vi "Parse EST Clusters into EST IP - Multi FPGA.vi"(8 "error in (no error)":errorcluster, 9 "RIO device address":string, 10 "EST version enum":T2, 11 "EPS IP LUT":variant) -> (0 "error out":errorcluster, 2 "Properties":T1[](array[typedef]), 3 "APUs":string[](array[string]))   [LabVIEW 2015, in "Engine Simulation Toolkit System Explorer.lvlib"]
uses:
  Engine Simulation Toolkit System Explorer.lvlib
  Shared/Bitfile EST Version.ctl
  String Array Property.ctl
  Shared/Properties.vi
  Shared/Engine Simulation Toolkit Shared.lvlib
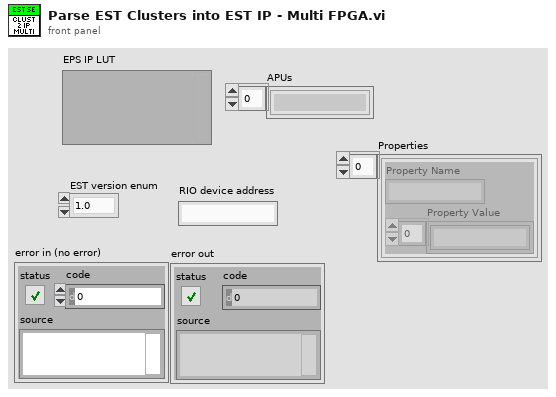
[diagram p1: front panel]
types:
  T1 = typedef "Engine Simulation Toolkit System Explorer.lvlib/String Array Property.ctl" = cluster{"Property Name":string, "Property Value":string[]}
  T2 = typedef "Engine Simulation Toolkit Shared.lvlib/Bitfile EST Version.ctl" = enum16{"1.0", "1.1", "1.2", "1.3"}
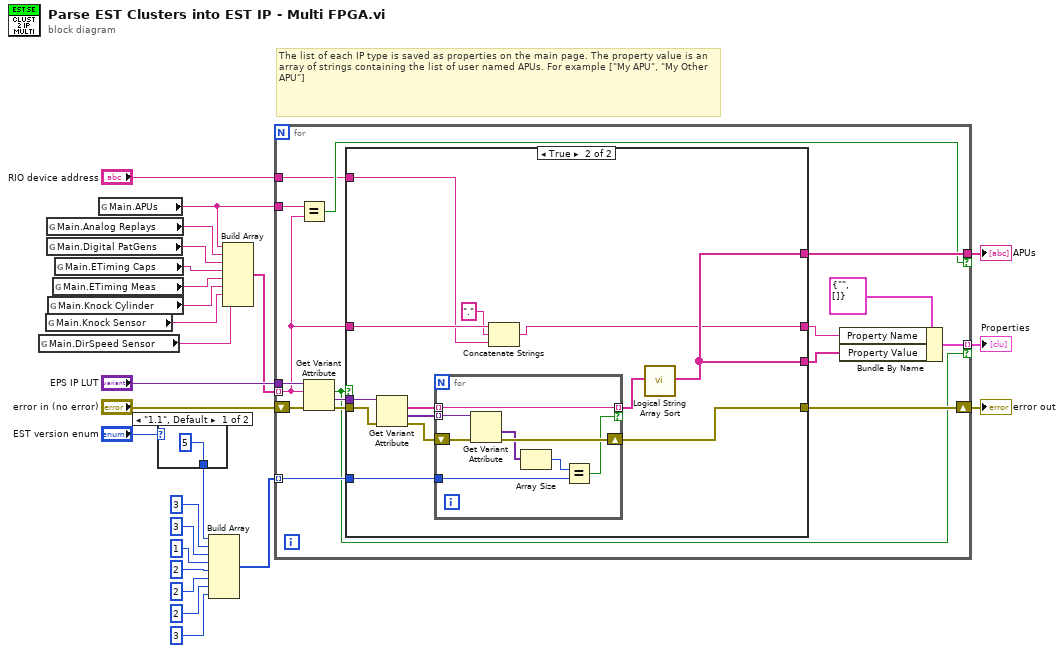
[diagram p0: block diagram]
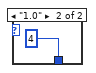
[diagram p2: hidden frame]
diagram:
  # "The list of each IP type is saved as properties on the main page. The property value is an array of strings containing the list of user named APUs. For example [\"My APU\", \"My Other APU\"]"
  n1 = global read "Properties.vi" "Main.DirSpeed Sensor"() -> (w5:string)
  n2 = global read "Properties.vi" "Main.Knock Sensor"() -> (w8:string)
  n3 = global read "Properties.vi" "Main.Analog Replays"() -> (w19:string)
  n4 = global read "Properties.vi" "Main.Digital PatGens"() -> (w18:string)
  n5 = global read "Properties.vi" "Main.Knock Cylinder"() -> (w9:string)
  n6 = global read "Properties.vi" "Main.ETiming Meas"() -> (w16:string)
  n7 = global read "Properties.vi" "Main.ETiming Caps"() -> (w17:string)
  n8 = global read "Properties.vi" "Main.APUs"() -> (w11:string)
  n9 = case shown="\"1.1\", Default" "EST version enum" {
    tunnel: [5 4] -> w20
    frame "1.1", Default {
    }
    frame "1.0" {
    }
  }
  n10 = Build Array(w20, 3, 3, 1, 2, 2, 2, 3) -> (w13:i32[])
  n11 = Build Array(w11, w19, w18, w17, w16, w9, w8, w5) -> (w14:string[])
  n12 = for {
    shift-right: [w39] -> w12
    shift-left: "error in (no error)" -> [w43]
    tunnel: "EPS IP LUT" -> [w42]
    tunnel: w14 -> [w37] mode=indexing
    tunnel: w13 -> [w38] mode=indexing
    tunnel: w11 -> [w36]
    tunnel: [w35] -> w10 if=w34
    tunnel: [w31] -> w2 mode=indexing if=w30
    tunnel: "RIO device address" -> [w28]
    n13 = Equal?(x=w36, y=w37) -> (x = y?=w34:bool)
    n14 = Get Variant Attribute(Variant=w42, name=w37, error in=w43) -> (found=w30:bool, value=w40:variant, error out=w41:errorcluster)  [unwired: 1 in, 1 out]
    n15 = case shown="True" w30 {
      tunnel: w41 -> [w45 w57]
      tunnel: w40 -> [_ w58]
      tunnel: [w45 w50] -> w39
      tunnel: w38 -> [_ w56]
      tunnel: w37 -> [w44 w49]
      tunnel: [_ w51] -> w35
      tunnel: [w44 w48] -> w33
      tunnel: [_ w51] -> w32
      tunnel: w28 -> [_ w46]
      frame False {
      }
      frame True {
        n16 = Get Variant Attribute(Variant=w58, error in=w57) -> (names=w54:string[], values=w53:variant[], error out=w55:errorcluster)  [unwired: 2 in, 1 out]
        n17 = for {
          tunnel: w56 -> [w66]
          shift-right: [w62] -> w50
          shift-left: w55 -> [w63]
          tunnel: w54 -> [w60] mode=indexing
          tunnel: w53 -> [w64] mode=indexing
          tunnel: [w60] -> w52 mode=indexing if=w59
          n18 = Get Variant Attribute(Variant=w64, error in=w63) -> (values=w61:variant[], error out=w62:errorcluster)  [unwired: 2 in, 2 out]
          n19 = Array Size(array=w61) -> (size(s)=w65:i32)
          n20 = Equal?(x=w65, y=w66) -> (x = y?=w59:bool)
        }
        n21 = Concatenate Strings(w49, "." ("string"), w46) -> (w48:string)
        n22 = call "Logical String Array Sort.vi"("Unsorted List"=w52) -> ("Sorted List"=w51:string[])  [unwired: 18 in]
      }
    }
    n23 = Bundle By Name(cluster=T1 {"Property Name"="", "Property Value"=[]} ("String Array Property"), "Property Name"=w33, "Property Value"=w32) -> (w31:T1)
  }
  "error out" <- w12
  "APUs" <- w10
  "Properties" <- w2
